vi "LineScanRemoteControl.vi"() -> ()   [LabVIEW 2022 SP3]
uses:
  Control_LineScanRemoteControl.ctl
  Control_LineScanCounterAE.ctl
  <vilib>/DAQmx/read.llb/DAQmx Read (Counter U32 1Chan 1Samp).vi
  <vilib>/DAQmx/create/channels.llb/DAQmx Create Channel (CI-Count Edges).vi
  <vilib>/DAQmx/miscellaneous.llb/DAQmx Fill In Error Info.vi
  <resource>/objmgr/daqmx.rc
panel:
  out "Last point\nduration (s)":dbl
  out "DAQ Errors":errorcluster={"status"=TRUE, "code"=-200088, "source"="DAQmx Stop Task.vi:3590007<append>\n"}
  out "Digital counter":u32
  in  "Trigger Edge":i32(ring)=10171 items=["Rising"=10280, "Falling"=10171]
  in  "Trigger Terminal":tag="PFI8"
  in  "TTL Control Active":bool
  out "Current point":i32
  out "Current\nAccumulation":i32
  in  "Finish point":bool
  in  "Next point":bool
  out "Linescan active":bool
  in  "Halt program":bool=TRUE
  in  "Stop linescan":bool
  in  "Start linescan":bool
  in  "Total # of Accumulations":i32=2
  in  "# of Points":i32=2 min=1 max=1000
  # "Linescan remote control"
  # "External TTL Control"
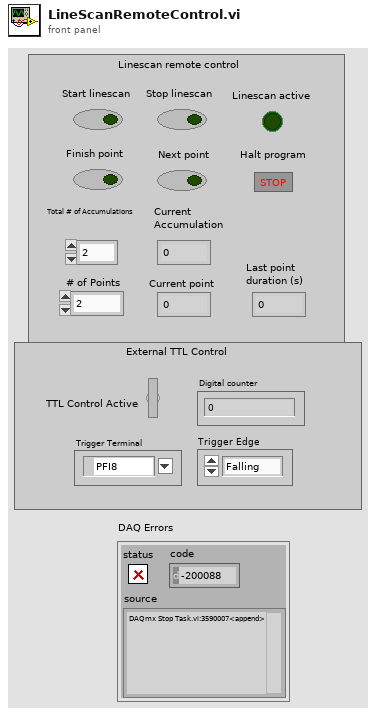
[diagram p1: front panel]
types:
  T1 = typedef "Control_LineScanRemoteControl.ctl" = enum16{"Start linescan", "Sit Idle", "Stop linescan", "Next Point", "Update from Counter", "Finish point", "Start DAQ control", "Poll DAQ control", "Stop DAQ control"}
  T2 = typedef "Control_LineScanCounterAE.ctl" = enum16{"Initialize", "Activate", "Attach indicators", "Increment Point", "Query", "Do Finish Point", "Acknowledge line", "Deactivate"}
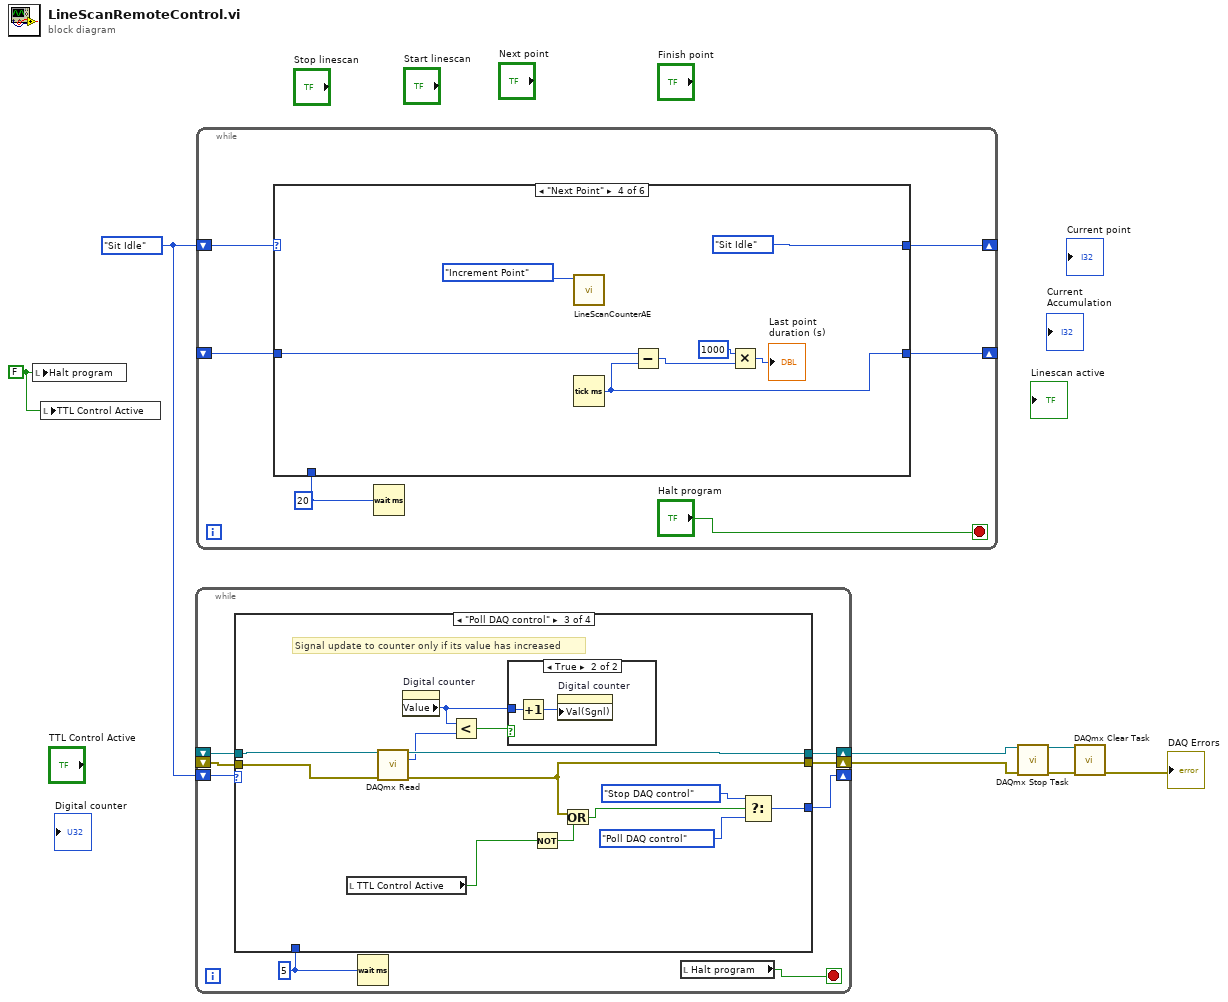
[diagram p0: block diagram]
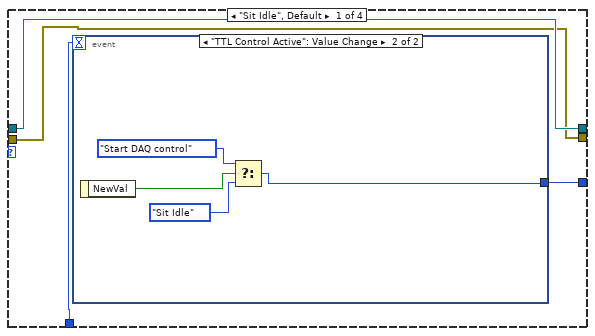
[diagram p2: hidden frame]
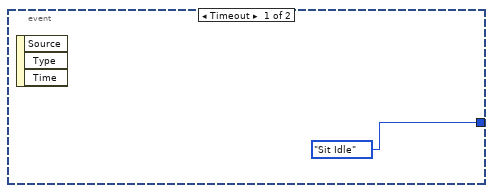
[diagram p3: hidden frame]
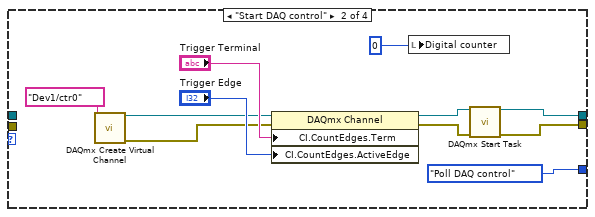
[diagram p4: hidden frame]
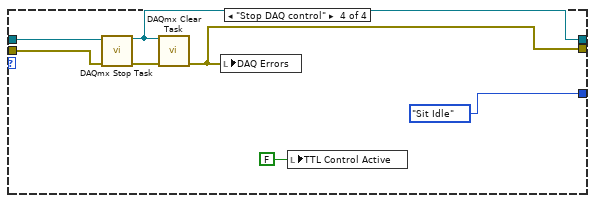
[diagram p6: hidden frame]
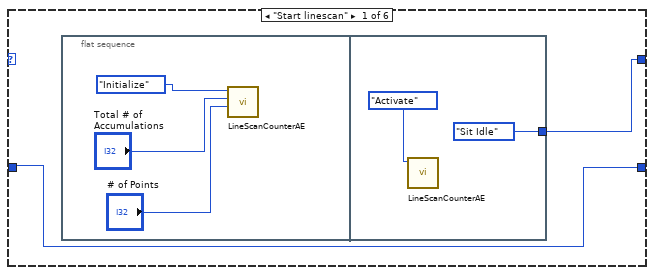
[diagram p7: hidden frame]
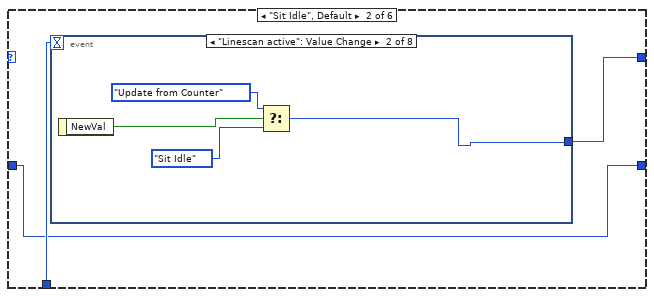
[diagram p8: hidden frame]
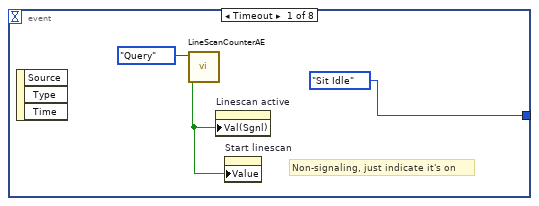
[diagram p9: hidden frame]
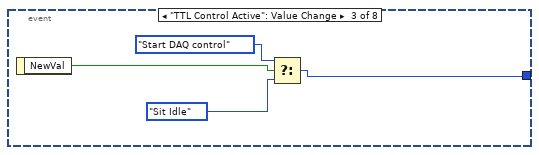
[diagram p10: hidden frame]
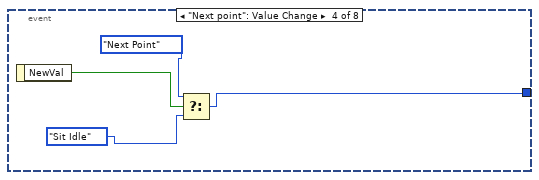
[diagram p11: hidden frame]
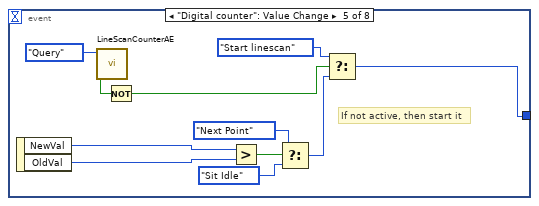
[diagram p12: hidden frame]
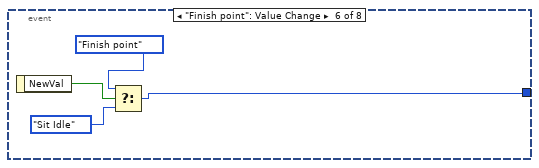
[diagram p13: hidden frame]
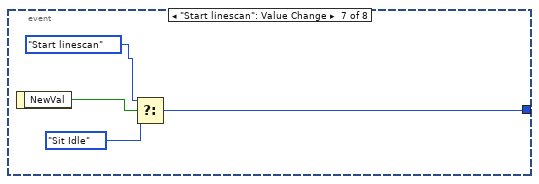
[diagram p14: hidden frame]
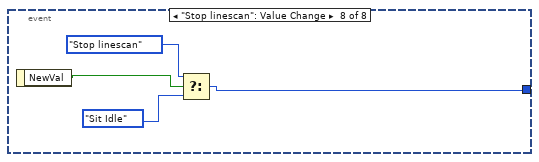
[diagram p15: hidden frame]
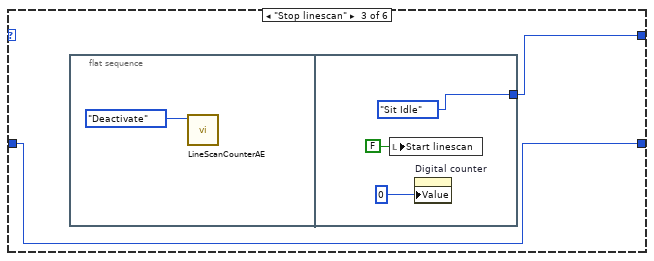
[diagram p16: hidden frame]
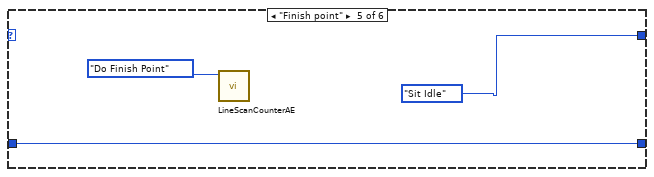
[diagram p17: hidden frame]
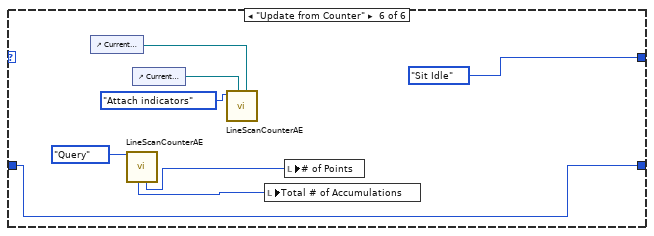
[diagram p18: hidden frame]
diagram:
  w1 = FALSE ("Halt program")
  w7 = Control_LineScanRemoteControl."Sit Idle"
  n1 = local write "Halt program"(w1) -> ()
  n2 = local write "TTL Control Active"(w1) -> ()
  n3 = while {
    shift-right: [w14] -> w4
    shift-left: _ -> [w12]
    shift-right: [w13] -> w3
    shift-left: _ -> [w11]
    shift-right: [w10] -> _
    shift-left: w7 -> [w15]
    stop <- w8 stop-if-true
    w9 = 5
    n4 = case shown="\"Poll DAQ control\"" w15 {
      tunnel: [w17 w26 w46 w53] -> w14
      tunnel: [w16 w25 w41 w52] -> w13
      tunnel: w12 -> [w17 _ w48 w56]
      tunnel: w11 -> [w16 _ w47 w55]
      tunnel: [w19 Control_LineScanRemoteControl."Poll DAQ control" w44 Control_LineScanRemoteControl."Sit Idle"] -> w10
      tunnel: w9 -> [w18 _ _ _]
      frame "Sit Idle", Default {
        n5 = event shown="[1] \"TTL Control Active\": Value Change" {
          selector: _ -> [_ _]
          dyn-events: _ -> [_ _]
          timeout: w18 -> [_ _]
          tunnel: [Control_LineScanRemoteControl."Sit Idle" w21] -> w19
          event Timeout {
            n6 = event-data() -> ()  [unwired: 1 in, 3 out]
          }
          event "TTL Control Active": Value Change {
            n7 = event-data() -> ("NewVal"=w24:bool)  [unwired: 1 in]
            n8 = Select(t=Control_LineScanRemoteControl."Start DAQ control", s=w24, f=Control_LineScanRemoteControl."Sit Idle") -> (s? t:f=w21:T1)
          }
        }
      }
      frame "Start DAQ control" {
        n9 = call-poly <vilib>:"DAQmx Create Virtual Channel.vi"("counter"=tag "Dev1/ctr0") -> ("task out"=w33:refnum<k21>, "error out"=w32:errorcluster)  [unwired: 13 in]
        n10 = property class="DAQmx Channel"(reference=w33, error in=w32, "CI.CountEdges.Term"="Trigger Terminal", "CI.CountEdges.ActiveEdge"="Trigger Edge") -> (reference out=w28:refnum<k21>, error out=w27:errorcluster)
        n11 = local write "Digital counter"(0) -> ()
        n12 = call <vilib>:"DAQmx Start Task.vi"("task/channels in"=w28, "error in"=w27) -> ("task out"=w26:refnum<k21>, "error out"=w25:errorcluster)  [unwired: 12 in]
      }
      frame "Poll DAQ control" {
        # "Signal update to counter only if its value has increased"
        n13 = local read "TTL Control Active"() -> (w39:bool)
        n14 = call-poly <vilib>:"DAQmx Read.vi"("task/channels in"=w48, "error in"=w47) -> ("task out"=w46:refnum<k21>, "data"=w38:u32, "error out"=w41:errorcluster)  [unwired: 11 in]
        n15 = property on="Digital counter" class="DigNum (strict)"() -> ("Value"=w37:u32)  [unwired: 2 in, 2 out]
        n16 = Less?(x=w37, y=w38) -> (x < y?=w36:bool)
        n17 = case shown="True" w36 {
          tunnel: w37 -> [_ w49]
          frame False {
          }
          frame True {
            n18 = Increment(x=w49) -> (x+1=w50:u32)
            n19 = property on="Digital counter" class="DigNum (strict)"("Val(Sgnl)"=w50) -> ()  [unwired: 2 in, 2 out]
          }
        }
        n20 = Not(x=w39) -> (.not. x?=w40:bool)
        n21 = Or(x=w41, y=w40) -> (x .or. y?=w42:bool)
        n22 = Select(t=Control_LineScanRemoteControl."Stop DAQ control", s=w42, f=Control_LineScanRemoteControl."Poll DAQ control") -> (s? t:f=w44:T1)
      }
      frame "Stop DAQ control" {
        n23 = call <vilib>:"DAQmx Stop Task.vi"("task/channels in"=w56, "error in"=w55) -> ("task out"=w53:refnum<k21>, "error out"=w57:errorcluster)  [unwired: 12 in]
        n24 = call <vilib>:"DAQmx Clear Task.vi"("task in"=w53, "error in"=w57) -> ("error out"=w52:errorcluster)  [unwired: 13 in]
        n25 = local write "DAQ Errors"(w52) -> ()
        n26 = local write "TTL Control Active"(FALSE ("DAQ Control Active")) -> ()
      }
    }
    n27 = Wait (ms)(milliseconds to wait=w9) -> ()  [unwired: 1 out]
    n28 = local read "Halt program"() -> (w8:bool)
  }
  n29 = while {
    shift-right: [w63] -> _
    shift-left: w7 -> [w60]
    shift-right: [w59] -> _
    shift-left: _ -> [w58]
    stop <- "Halt program" stop-if-true
    w61 = 20
    n30 = case shown="\"Next Point\"" w60 {
      tunnel: [w65 w72 w113 Control_LineScanRemoteControl."Sit Idle" Control_LineScanRemoteControl."Sit Idle" Control_LineScanRemoteControl."Sit Idle"] -> w63
      tunnel: w61 -> [_ w73 _ _ _ _]
      tunnel: [w64 w71 w112 w122 w125 w128] -> w59
      tunnel: w58 -> [w64 w71 w112 w121 w125 w128]
      frame "Start linescan" {
        n31 = flat-sequence {
          tunnel: [Control_LineScanRemoteControl."Sit Idle"] -> w65
          frame #0 {
            n32 = call "LineScanCounterAE.vi"("Number of points"="# of Points", "Accumulate to #"="Total # of Accumulations", "Task"=Control_LineScanCounterAE."Initialize" ("Enum")) -> ()  [unwired: 2 in, 7 out]
          }
          frame #1 {
            n33 = call "LineScanCounterAE.vi"("Task"=Control_LineScanCounterAE."Activate" ("Enum")) -> ()  [unwired: 4 in, 7 out]
          }
        }
      }
      frame "Sit Idle", Default {
        n34 = event shown="[1] \"Linescan active\": Value Change" {
          selector: _ -> [_ _ _ _ _ _ _ _]
          dyn-events: _ -> [_ _ _ _ _ _ _ _]
          timeout: w73 -> [_ _ _ _ _ _ _ _]
          tunnel: [Control_LineScanRemoteControl."Sit Idle" w77 w81 w87 w92 w102 w106 w110] -> w72
          event Timeout {
            # "Non-signaling, just indicate it's on"
            n35 = event-data() -> ()  [unwired: 1 in, 3 out]
            n36 = call "LineScanCounterAE.vi"("Task"=Control_LineScanCounterAE."Query" ("Enum")) -> ("Active"=w74:bool)  [unwired: 4 in, 6 out]
            n37 = property on="Linescan active" class="Bool (strict)"("Val(Sgnl)"=w74) -> ()  [unwired: 2 in, 2 out]
            n38 = property on="Start linescan" class="Bool (strict)"("Value"=w74) -> ()  [unwired: 2 in, 2 out]
          }
          event "Linescan active": Value Change {
            n39 = event-data() -> ("NewVal"=w78:bool)  [unwired: 1 in]
            n40 = Select(t=Control_LineScanRemoteControl."Update from Counter", s=w78, f=Control_LineScanRemoteControl."Sit Idle") -> (s? t:f=w77:T1)
          }
          event "TTL Control Active": Value Change {
            n41 = event-data() -> ("NewVal"=w82:bool)  [unwired: 1 in]
            n42 = Select(t=Control_LineScanRemoteControl."Start DAQ control", s=w82, f=Control_LineScanRemoteControl."Sit Idle") -> (s? t:f=w81:T1)
          }
          event "Next point": Value Change {
            n43 = event-data() -> ("NewVal"=w88:bool)  [unwired: 1 in]
            n44 = Select(t=Control_LineScanRemoteControl."Next Point", s=w88, f=Control_LineScanRemoteControl."Sit Idle") -> (s? t:f=w87:T1)
          }
          event "Digital counter": Value Change {
            # "If not active, then start it"
            n45 = event-data() -> ("NewVal"=w95:u32, "OldVal"=w98:u32)  [unwired: 1 in]
            n46 = call "LineScanCounterAE.vi"("Task"=Control_LineScanCounterAE."Query" ("Enum")) -> ("Active"=w90:bool)  [unwired: 4 in, 6 out]
            n47 = Not(x=w90) -> (.not. x?=w89:bool)
            n48 = Greater?(x=w95, y=w98) -> (0:w97:bool)
            n49 = Select(t=Control_LineScanRemoteControl."Next Point", s=w97, f=Control_LineScanRemoteControl."Sit Idle") -> (s? t:f=w93:T1)
            n50 = Select(t=Control_LineScanRemoteControl."Start linescan", s=w89, f=w93) -> (s? t:f=w92:T1)
          }
          event "Finish point": Value Change {
            n51 = event-data() -> ("NewVal"=w103:bool)  [unwired: 1 in]
            n52 = Select(t=Control_LineScanRemoteControl."Finish point", s=w103, f=Control_LineScanRemoteControl."Sit Idle") -> (s? t:f=w102:T1)
          }
          event "Start linescan": Value Change {
            n53 = event-data() -> ("NewVal"=w107:bool)  [unwired: 1 in]
            n54 = Select(t=Control_LineScanRemoteControl."Start linescan", s=w107, f=Control_LineScanRemoteControl."Sit Idle") -> (s? t:f=w106:T1)
          }
          event "Stop linescan": Value Change {
            n55 = event-data() -> ("NewVal"=w111:bool)  [unwired: 1 in]
            n56 = Select(t=Control_LineScanRemoteControl."Stop linescan", s=w111, f=Control_LineScanRemoteControl."Sit Idle") -> (s? t:f=w110:T1)
          }
        }
      }
      frame "Stop linescan" {
        n57 = flat-sequence {
          tunnel: [Control_LineScanRemoteControl."Sit Idle"] -> w113
          frame #0 {
            n58 = call "LineScanCounterAE.vi"("Task"=Control_LineScanCounterAE."Deactivate" ("Enum")) -> ()  [unwired: 4 in, 7 out]
          }
          frame #1 {
            n59 = local write "Start linescan"(FALSE ("Start linescan")) -> ()
            n60 = property on="Digital counter" class="DigNum (strict)"("Value"=0) -> ()  [unwired: 2 in, 2 out]
          }
        }
      }
      frame "Next Point" {
        n61 = call "LineScanCounterAE.vi"("Task"=Control_LineScanCounterAE."Increment Point" ("Enum")) -> ()  [unwired: 4 in, 7 out]
        n62 = Tick Count (ms)() -> (millisecond timer value=w122:u32)
        n63 = Subtract(x=w121, y=w122) -> (x-y=w119:u32)
        n64 = Multiply(x=1000, y=w119) -> (x*y=→"Last point\nduration (s)":u32)
      }
      frame "Finish point" {
        n65 = call "LineScanCounterAE.vi"("Task"=Control_LineScanCounterAE."Do Finish Point" ("Enum")) -> ()  [unwired: 4 in, 7 out]
      }
      frame "Update from Counter" {
        n66 = control-ref of="Current\nAccumulation"() -> (w130:refnum<vi>)
        n67 = call "LineScanCounterAE.vi"("Task"=Control_LineScanCounterAE."Query" ("Enum")) -> ("Number of points (query)"=w134:i32, "Accumulate to (query)"=w133:i32)  [unwired: 4 in, 5 out]
        n68 = control-ref of="Current point"() -> (w135:refnum<vi>)
        n69 = call "LineScanCounterAE.vi"("# Accumulated (reference)"=w130, "Current point index (reference)"=w135, "Task"=Control_LineScanCounterAE."Attach indicators" ("Enum")) -> ()  [unwired: 2 in, 7 out]
        n70 = local write "Total # of Accumulations"(w133) -> ()
        n71 = local write "# of Points"(w134) -> ()
      }
    }
    n72 = Wait (ms)(milliseconds to wait=w61) -> ()  [unwired: 1 out]
  }
  n73 = call <vilib>:"DAQmx Stop Task.vi"("task/channels in"=w4, "error in"=w3) -> ("task out"=w5:refnum<k21>, "error out"=w6:errorcluster)  [unwired: 12 in]
  n74 = call <vilib>:"DAQmx Clear Task.vi"("task in"=w5, "error in"=w6) -> ("error out"=→"DAQ Errors":errorcluster)  [unwired: 13 in]
